vi "STA - Wave V5 Host_Wait_V2.vi"() -> ()   [LabVIEW 2015]
doc: "The continuous acquisition mode tells the FPGA to acquire points indefinitely until a stop command is issued or until an error is encountered (FIFO overflow, module underflow, and so on). \n\nIn this acquisition mode, explicitly call the appropriate rwfm_ConfigTiming VI and set the host application's data buffer to be many times larger than the read size. The examples use a 10X size by default. If the host application's data buffer fills, then the FPGA experiences a FIFO overflow causing the acquisition to stop."
uses:
  <vilib>/LabVIEW Targets/FPGA/cRIO/shared/nicrio_ModuleControls/nicrio_cRIO-9234_ConfigModeRing.ctl
  <vilib>/Platform/TimedLoop/XDataNode/timing_clust.ctl
  <vilib>/Platform/TimedLoop/XDataNode/nitl_modes.ctl
  <vilib>/Platform/TimedLoop/XDataNode/wakeup.ctl
  <vilib>/FPGAPlugInAG/cRIO-9112/niLvFpga_Open_cRIO-9112.vi
  <vilib>/rvi/interface/common/dynamic/niFpgaDynamicAddResources.vi
  <vilib>/Utility/error.llb/Error Cluster From Error Code.vi
  <vilib>/RVI Host/nirviSupport.llb/nirviErrorClusterFromErrorCode.vi
  <vilib>/rvi/errors/niLvFpgaAdjustHostInterfaceError.vi
  <vilib>/FPGAPlugInAG/Dynamic/niLvFpga_Close_Dynamic.vi
  <vilib>/rvi/interface/nirviOpenFPGA/nirviOpenFPGA.xnode
  FPGA Bitfiles/STA-WaveformV5_FPGATarget2_[FPGA]DeltaSigMa_sLRIAVfzKK0.lvbitx
  FPGA/[FPGA] DeltaSig Main V5.vi
  <vilib>/rvi/interface/nirviMethod/nirviMethod.xnode
  <vilib>/rvi/interface/nirviCloseFPGA/nirviCloseFPGA.xnode
  <vilib>/Platform/TimedLoop/XDataNode/XDataNode.xnode
  <vilib>/NI/cRIO Wfm/cRIO Wfm.lvlib
  <vilib>/rvi/interface/nirviMethod/StockFPGA_InlinedMethodWaitForSingleIRQ.vi
  <vilib>/FPGAPlugInAG/Dynamic/niLvFpga_WaitOnIrq_Dynamic.vi
  C:/Program Files (x86)/National Instruments/LabVIEW 2015/ProjectTemplates/Source/cRIOWfm/FPGA/[FPGA] SAR Acq Main.vi
  D/Documents/LabVIEW Data/STA - Waveform V0/FPGA Bitfiles/SARAcqMain_9074.lvbitx
  <vilib>/Platform/TimedLoop/XDataNode/XDNodeRunTimeDep.lvlib
panel:
  in  "transposed array 2":sgl[][](array[numeric])
  out "transposed array":sgl[][](array[numeric])
  out "error out 2":errorcluster
  out "error out":errorcluster
  out "error fifo out":errorcluster
  out "Waveform Graph 2":waveform(sgl)[](graph)
  in  "Array":waveform(sgl)[](array[waveform])
  out "Waveform Graph":waveform(sgl)[](graph)
  out "Buffer Backlog":dbl caption="RT Buffer Backlog [%]" format="%#.2g"
  in  "Stop":bool
  in  "Amplitude":dbl(slide)=5.0 scale=0.0..10.0
  out "Time Measure":dbl
  out "data rate (S/s)":u32
  out "Channel Config":T2(array[cluster]) {"Input Configuration" items=["AC Coupled", "DC Coupled", "IEPE AC Coupled"]}
  in  "Samples per Read":i32=900
  # "Sampling Info"
  # "Channel Info"
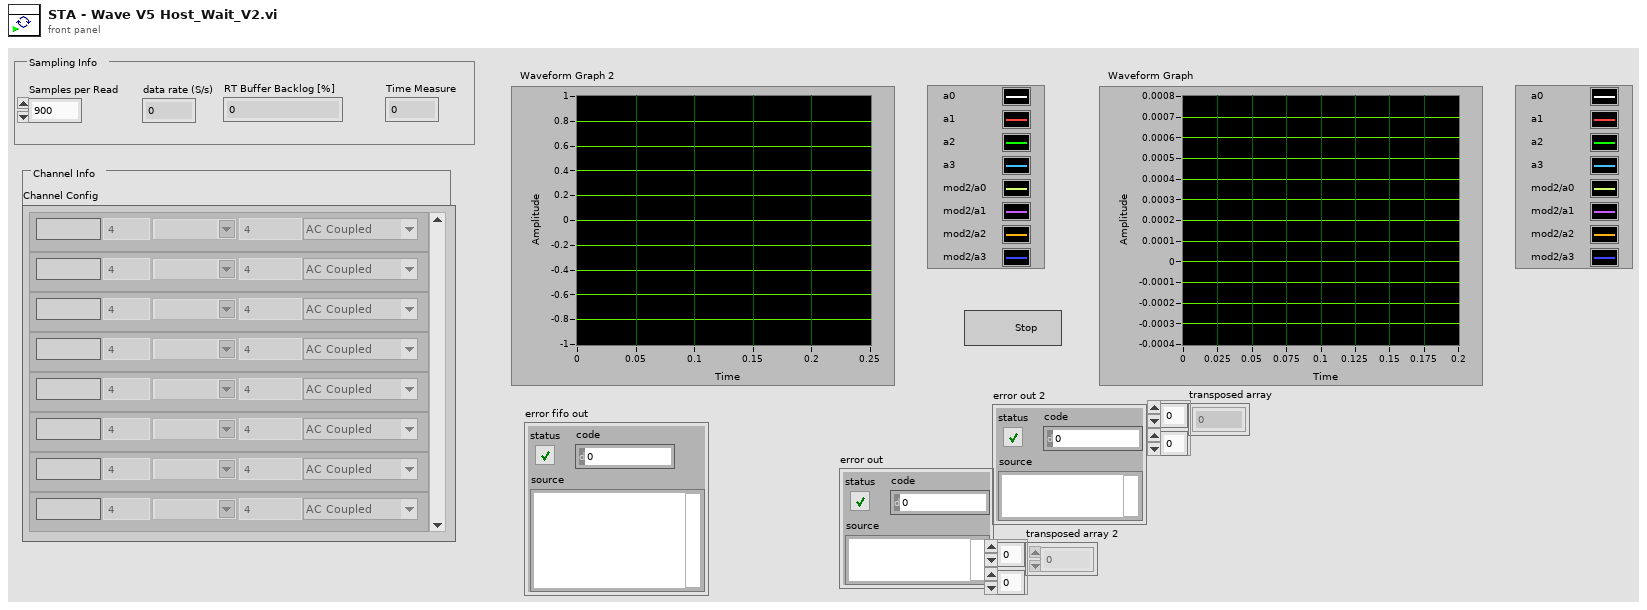
[diagram p1: front panel]
types:
  T1 = typedef "nicrio_cRIO-9234_ConfigModeRing.ctl" = u8
  T2 = cluster{"Channel Name":string, "Sensitivity mV_EU":dbl, "EU":string, "Input Configuration":T1, "dB Ref EU":dbl}[]
  T3 = typedef "XDNodeRunTimeDep.lvlib/timing_clust.ctl" = cluster{"Expected End [f-1]":u64, "Actual End [f-1]":u64, "Finished Late? [f-1]":bool, "Expected End [i-1]":u64, "Actual End [i-1]":u64, "Finished Late? [i-1]":bool, "Expected Start [i]":u64, "Actual Start [i]":u64, "Expected Start [f]":u64, "Actual Start [f]":u64, "Source Name":string, "Structure Name":string, "Period":i64, "Deadline":i64, "Offset":i64, "Start":i64, "Priority":i32, "Timeout":i32, "Mode":T4, "Wakeup Reason":T5, "Error":errorcluster, "Source Type":string, "Secondary Source Type":string, "Global End Time":u64, "Global Start Time":u64, "Frame Duration":u64, "Iteration Duration":u64, "Assigned CPU":i32, "I/O Scan Engine Mode":u32}
  T4 = typedef "XDNodeRunTimeDep.lvlib/nitl_modes.ctl" = enum32{"No Change", "Process missed periods, maintain original phase", "Discard missed periods, maintain original phase", "Process missed periods, ignore original phase", "Discard missed periods, ignore original phase"}
  T5 = typedef "XDNodeRunTimeDep.lvlib/wakeup.ctl" = enum32{"Normal", "Aborted", "Asynchronous wakeup", "Timing source error", "Timed loop error", "Timeout"}
  T6 = typedef "Acquisition and Logging Configuration_Waveform.ctl" = cluster{"Data Rate":T7, "Samples per Read":i32, "Number of Reads to Save":i32, "Data File Name":string, "TDMS Properties":T8[], "Number of Channels":i32, "Trigger - RMS Value":dbl, "Trigger - Channel":i32, "Trigger - Time (Minute)":i32, "Channel Config":cluster{"Channel Name":string, "Sensitivity mV_EU":dbl, "EU":string, "Input Configuration":T1, "dB Ref EU":dbl}[], "data rate (S/s)":u32, "Time Measure":dbl}
  T7 = typedef "nicrio_cRIO-9234_DataRatesRing2.ctl" = u8
  T8 = typedef "TDMS Properties.ctl" = cluster{"Name":string, "Value":string}
  T9 = typedef "cRIO Wfm.lvlib/SamplingInfo.ctl" = cluster{"Number of Channels":i32, "Actual Samp Rate":dbl, "Chan Name Array":string[], "EU Chan Array":string[], "dB Ref Chan Array":dbl[]}
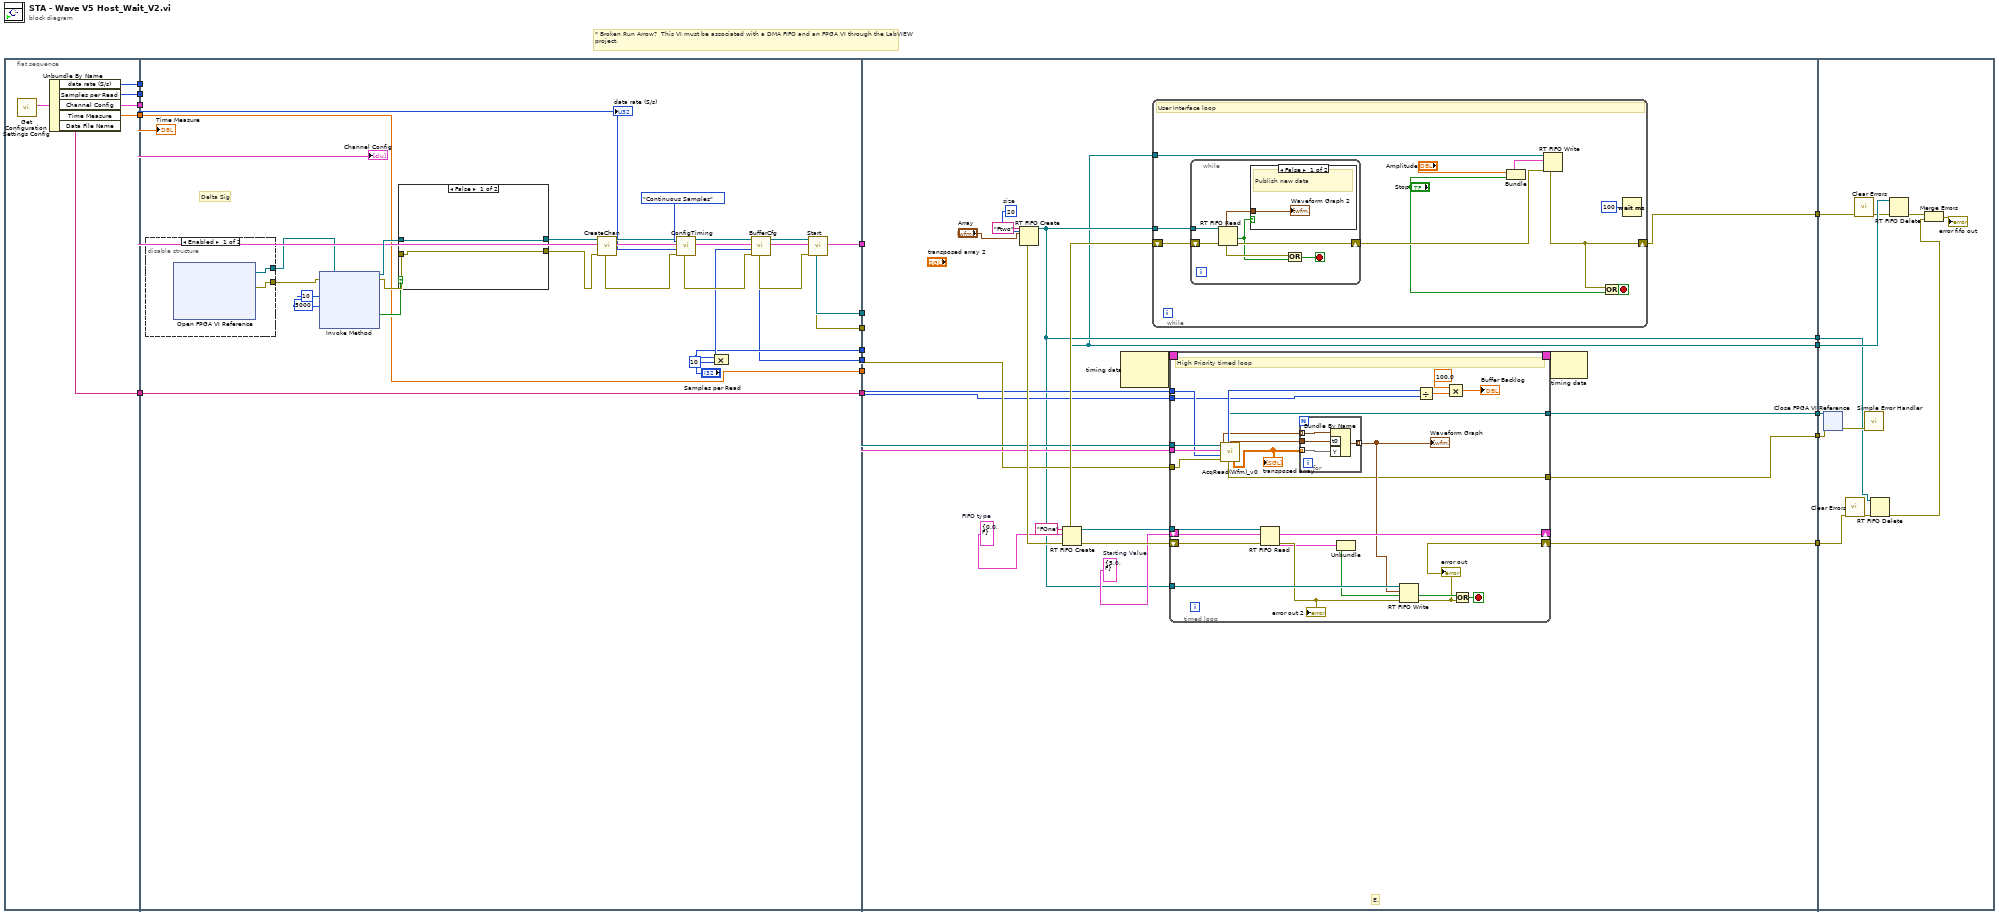
[diagram p0: block diagram]
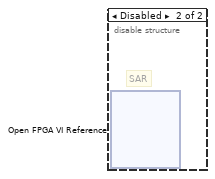
[diagram p2: hidden frame]
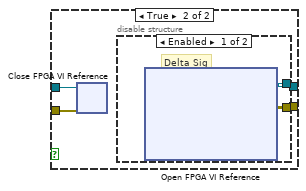
[diagram p3: hidden frame]
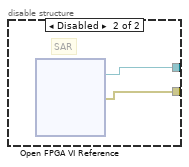
[diagram p4: hidden frame]
diagram:
  # "* Broken Run Arrow?  This VI must be associated with a DMA FIFO and an FPGA VI through the LabVIEW project."
  n1 = flat-sequence {
    tunnel: [w23] -> w18
    tunnel: [w22] -> w17
    tunnel: [w21] -> w16
    tunnel: [w20] -> w15
    tunnel: [w19] -> w8
    tunnel: w18 -> [w36]
    tunnel: w17 -> [_]
    tunnel: w16 -> [w35]
    tunnel: w15 -> [w28]
    tunnel: ["Samples per Read"] -> w14
    tunnel: [w28] -> w13
    tunnel: [w32] -> w12
    tunnel: [w31] -> w11
    tunnel: [w30] -> w10
    tunnel: [w27] -> w9
    tunnel: w8 -> [w26]
    tunnel: [w26] -> w7
    tunnel: w14 -> [w79]
    tunnel: w13 -> [_]
    tunnel: w12 -> [w81]
    tunnel: w11 -> [w82]
    tunnel: w10 -> [w80]
    tunnel: w9 -> [w78]
    tunnel: w7 -> [_]
    tunnel: [w75] -> w6
    tunnel: [w74] -> w5
    tunnel: [w73] -> w4
    tunnel: [w72] -> w3
    tunnel: [w71] -> w2
    tunnel: [w70] -> w1
    tunnel: w6 -> [w146]
    tunnel: w5 -> [w145]
    tunnel: w4 -> [w144]
    tunnel: w3 -> [w142]
    tunnel: w2 -> [w143]
    tunnel: w1 -> [w141]
    frame #0 {
      n2 = call "Get Configuration Settings Config.vi"() -> ("Configuration"=w24:T6)  [unwired: 10 in, 1 out]
      n3 = Unbundle By Name(w24) -> ("data rate (S/s)"=w23:u32, "Samples per Read"=w22:i32, "Channel Config"=w21:T2, "Time Measure"=w20:dbl, "Data File Name"=w19:string)
    }
    frame #1 {
      # "Delta Sig"
      n4 = disable-structure shown="Enabled" {
        disable-tunnel: [w56 _] -> w34
        disable-tunnel: [w55 _] -> w33
        frame Enabled {
          n5 = xnode "Open FPGA VI Reference"() -> ("FPGA VI Reference Out"=w56:refnum<k20>, "error out"=w55:errorcluster)  [unwired: 2 in]
        }
        frame Disabled {
          # "SAR"
          n6 = xnode "Open FPGA VI Reference"() -> ("FPGA VI Reference Out"=w58:refnum<k20>, "error out"=w57:errorcluster)  [unwired: 2 in]
        }
      }
      n7 = xnode "Invoke Method"("FPGA VI Reference In"=w34, "error in"=w33, "IRQ Number(s)"=10, "Timeout (ms)"=5000) -> ("FPGA VI Reference Out"=w52:refnum<k20>, "error out"=w53:errorcluster, "Timed Out"=w51:bool)  [unwired: 1 out]
      n8 = case shown="False" w51 {
        tunnel: w52 -> [w60 w64]
        tunnel: w53 -> [w59 w63]
        tunnel: [w60 w62] -> w25
        tunnel: [w59 w61] -> w54
        frame False {
        }
        frame True {
          n9 = xnode "Close FPGA VI Reference"("FPGA VI Reference In"=w64, "error in"=w63) -> ()  [unwired: 1 out]
          n10 = disable-structure shown="Enabled" {
            disable-tunnel: [w66 w68] -> w62
            disable-tunnel: [w65 w67] -> w61
            frame Enabled {
              # "Delta Sig"
              n11 = xnode "Open FPGA VI Reference"() -> ("FPGA VI Reference Out"=w66:refnum<k20>, "error out"=w65:errorcluster)  [unwired: 2 in]
            }
            frame Disabled {
              # "SAR"
              n12 = xnode "Open FPGA VI Reference"() -> ("FPGA VI Reference Out"=w68:refnum<k20>, "error out"=w67:errorcluster)  [unwired: 2 in]
            }
          }
        }
      }
      n13 = call <vilib>:"CreateChan.vi"("Dynamic FPGA Ref"=w25, "Channel Config"=w35, "error in"=w54) -> ("Dynamic FPGA Ref Out"=w42:refnum<k20>, "Sampling Info"=w43:T9, "error out"=w47:errorcluster)  [unwired: 5 in]
      n14 = call <vilib>:"ConfigTiming.vi"("Sample Mode"=enum16{"Finite Samples", "Continuous Samples"}."Continuous Samples", "error in"=w47, "Sample Rate"=w36, "Sampling Info In"=w43, "Dynamic FPGA Ref"=w42) -> ("error out"=w46:errorcluster, "Sampling Info Out"=w45:T9, "Dynamic FPGA Ref Out"=w44:refnum<k20>)  [unwired: 3 in, 1 out]
      n15 = Compound Arithmetic op=MULTIPLY("Samples per Read", 10 ("value")) -> (w40:i32)
      n16 = call <vilib>:"BufferCfg.vi"("error in"=w46, "Buffer Size [Samps per Chan]"=w40, "Sampling Info In"=w45, "Dynamic FPGA Ref"=w44) -> ("error out"=w39:errorcluster, "Buffer Size [Total Samples]"=w27:u32, "Sampling Info Out"=w41:T9, "Dynamic FPGA Ref Out"=w38:refnum<k20>)  [unwired: 4 out]
      n17 = call <vilib>:"Start.vi"("error in"=w39, "Sampling Info In"=w41, "Dynamic FPGA Ref"=w38) -> ("error out"=w30:errorcluster, "Sampling Info Out"=w31:T9, "Dynamic FPGA Ref Out"=w32:refnum<k20>)  [unwired: 6 out]
      "Channel Config" <- w35
      "data rate (S/s)" <- w36
      "Time Measure" <- w28
    }
    frame #2 {
      w83 = cluster{dbl, bool} {5.0, FALSE}  # Starting Value
      w84 = cluster{dbl, bool} {0.0, FALSE}  # FIFO type
      w85 = u32 20  # size
      # "E."
      n18 = RT FIFO Create(0:"Ftwo" ("name (unnamed)"), 1:"Array", 4:w85) -> (8:w72:refnum<k33>, 11:w87:errorcluster)  [unwired: 2 in, 4 out]
      n19 = RT FIFO Create(0:"FOne" ("name (unnamed)"), 1:w84, 3:w87) -> (8:w71:refnum<k33>, 11:w86:errorcluster)  [unwired: 2 in, 4 out]
      n20 = node-c288() -> (w89:T3)  [unwired: 1 in, 1 out]
      n21 = while "User Interface loop" {
        shift-right: [w90] -> w70
        shift-left: w86 -> [w98]
        tunnel: w71 -> [w97]
        tunnel: w72 -> [w99]
        stop <- w95 stop-if-true
        # "User Interface loop"
        n22 = while {
          tunnel: w99 -> [w105]
          shift-right: [w101] -> w96
          shift-left: w98 -> [w104]
          stop <- w102 stop-if-true
          n23 = RT FIFO Read(0:w105, 3:w104) -> (9:w103:waveform(sgl)[], 10:w100:bool, 11:w101:errorcluster)  [unwired: 1 in, 3 out]
          n24 = case shown="False" w100 {
            tunnel: w103 -> [w106 _]
            frame False {
              # "Publish new data"
              "Waveform Graph 2" <- w106
            }
            frame True {
              # "No new data"
            }
          }
          n25 = Or(x=w101, y=w100) -> (x .or. y?=w102:bool)
        }
        n26 = Bundle("Amplitude"="Amplitude", "Stop"="Stop") -> (w92:cluster{"Amplitude":dbl, "Stop":bool})  [unwired: 1 in]
        n27 = RT FIFO Write(0:w97, 1:w92, 3:w96) -> (11:w90:errorcluster)  [unwired: 2 in, 3 out]
        n28 = Or(x=w90, y="Stop") -> (x .or. y?=w95:bool)
        n29 = Wait (ms)(milliseconds to wait=u32 100 ("millisecond multiple")) -> ()  [unwired: 1 out]
      }
      n30 = timed-loop "High Priority timed loop" {
        shift-left: w83 -> [w129]
        shift-right: [w125] -> _
        shift-right: [w107] -> w73
        shift-left: w86 -> [w126]
        timing: w89 -> [_]
        timing-out: [_] -> w88
        tunnel: w71 -> [w130]
        tunnel: w72 -> [w128]
        tunnel: w82 -> [w116]
        tunnel: w81 -> [w115]
        tunnel: w80 -> [w114]
        tunnel: w79 -> [w112]
        tunnel: w78 -> [w111]
        tunnel: [w109] -> w75
        tunnel: [w108] -> w74
        stop <- w123 stop-if-true
        # "High Priority timed loop"
        n31 = call <vilib>:"AcqRead(Wfm)_v0.vi"("error in"=w114, "Samps Read per Chan"=w112, "Sampling Info"=w116, "Dynamic FPGA Ref"=w115) -> ("error out"=w108:errorcluster, "Samples Remaining"=w122:u32, "time stamp"=w117:timestamp, "Dynamic FPGA Ref Out"=w109:refnum<k20>, "transposed array"=w113:sgl[][], "Array"=w118:waveform(sgl)[])  [unwired: 2 in]
        "transposed array" <- w113
        n32 = RT FIFO Read(0:w130, 1:w129, 3:w126) -> (9:w125:cluster{dbl, bool}, 11:w127:errorcluster)  [unwired: 4 out]
        "error out 2" <- w127
        n33 = for {
          tunnel: w118 -> [w134] mode=indexing
          tunnel: w117 -> [w133]
          tunnel: [w132] -> w110 mode=indexing
          tunnel: w113 -> [w131] mode=indexing
          n34 = Bundle By Name(cluster=w134, "t0"=w133, "Y"=w131) -> (w132:waveform(sgl))
        }
        "Waveform Graph" <- w110
        n35 = Unbundle(w125) -> (w124:bool)  [unwired: 1 out]
        n36 = RT FIFO Write(0:w128, 1:w110, 3:w127) -> (11:w107:errorcluster)  [unwired: 1 in, 4 out]
        "error out" <- w107
        n37 = Divide(x=w122, y=w111) -> (x/y=w121:dbl)
        n38 = Multiply(x=100.0, y=w121) -> (x*y=→"Buffer Backlog":dbl)
        n39 = Or(x=w124, y=w107) -> (x .or. y?=w123:bool)
      }
      n40 = node-c288(w88) -> ()  [unwired: 1 out]
    }
    frame #3 {
      n41 = xnode "Close FPGA VI Reference"("FPGA VI Reference In"=w146, "error in"=w145) -> ("error out"=w150:errorcluster)
      n42 = call <vilib>:"Clear Errors.vi"("error in (no error)"=w144) -> ("error out"=w147:errorcluster)  [unwired: 5 in, 1 out]
      n43 = call <vilib>:"Clear Errors.vi"("error in (no error)"=w141) -> ("error out"=w140:errorcluster)  [unwired: 5 in, 1 out]
      n44 = call <vilib>:"Simple Error Handler.vi"("error in (no error)"=w150) -> ()  [unwired: 1 in, 8 out]
      n45 = RT FIFO Delete(0:w142, 3:w147) -> (11:w139:errorcluster)  [unwired: 1 in]
      n46 = RT FIFO Delete(0:w143, 3:w140) -> (11:w148:errorcluster)  [unwired: 1 in]
      n47 = Merge Errors(w148, w139) -> (→"error fifo out":errorcluster)
    }
  }
